vi "Init JSON Config File.vi"(8 "error in (no error)":errorcluster, 10 "Path":path, 11 "JSON Config File in":refnum<class "JSON Config File.lvclass">) -> (0 "error out":errorcluster, 3 "JSON Config File out":refnum<class "JSON Config File.lvclass">)   [LabVIEW 2013, in "JSON Config File.lvclass"]
uses:
  JSON Config File.lvclass
  JSON Config File.lvclass/JSON Config File.ctl
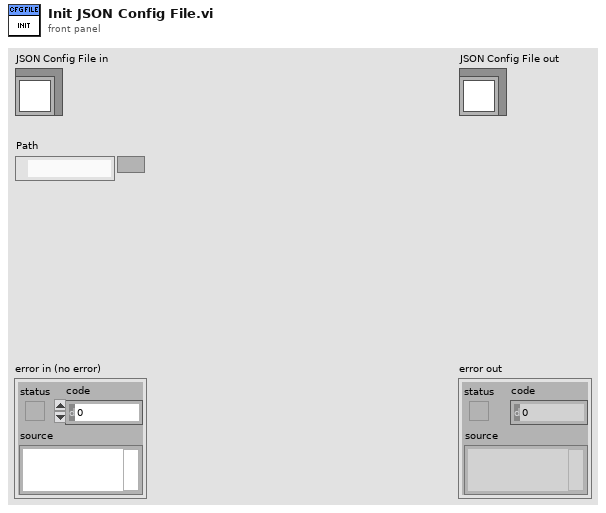
[diagram p1: front panel]
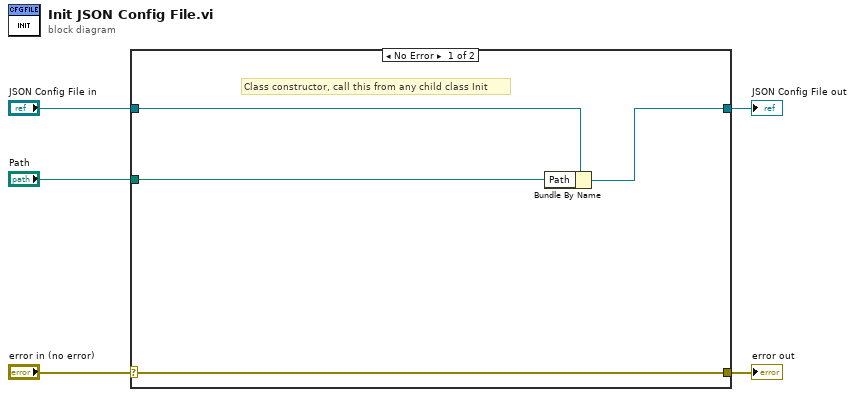
[diagram p0: block diagram]
diagram:
  n1 = case shown="No Error" "error in (no error)" {
    selector: "error in (no error)" -> [w9 w11]
    tunnel: [w9 w11] -> w4
    tunnel: [w7 w10] -> w2
    tunnel: "JSON Config File in" -> [w8 w10]
    tunnel: "Path" -> [w6 _]
    frame No Error {
      # "Class constructor, call this from any child class Init"
      n2 = Bundle By Name(cluster=w8, "Path"=w6) -> (w7:refnum<class "JSON Config File.lvclass">)
    }
    frame Error {
    }
  }
  "error out" <- w4
  "JSON Config File out" <- w2
